vi "BeamGage Callback with notification.vi"(4 "User Parameter":T1, 6 "Control Ref":refnum<k24>, 7 "Event Common Data":T2) -> ()   [LabVIEW 2011]
doc: "A .net callback VI that queries BeamGage for Divergence measurements. Divergence results are loaded into a notifier queue than can be read by an upper level VI as new results become available."
uses:
  C:/Program Files/Spiricon/BeamGage Professional/Spiricon.BeamGage.Automation.Interfaces.dll
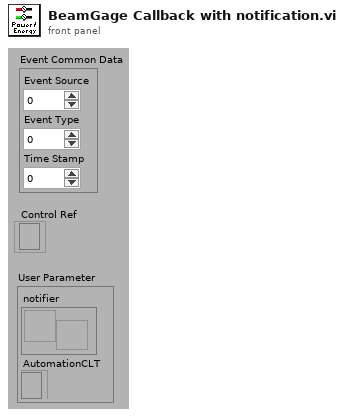
[diagram p1: front panel]
types:
  T1 = cluster{"notifier":refnum<notifier>, "AutomationCLT":refnum<k24>}
  T2 = cluster{"Event Source":i32, "Event Type":u32, "Time Stamp":u32}
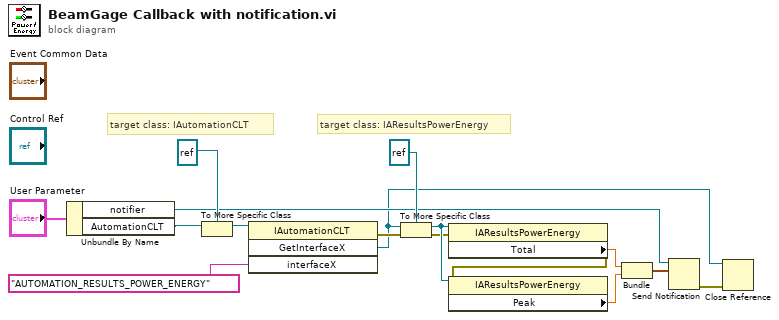
[diagram p0: block diagram]
diagram:
  # "target class: IAResultsPowerEnergy"
  # "target class: IAutomationCLT"
  n1 = Unbundle By Name("User Parameter") -> ("notifier"=w3:refnum<notifier>, "AutomationCLT"=w9:refnum<k24>)
  n2 = To More Specific Class(target class=refnum<k24> refnum, reference=w9) -> (specific class reference=w8:refnum<k24>)  [unwired: 1 in, 1 out]
  n3 = invoke class="IAutomationCLT" method="GetInterfaceX"(reference=w8, "interfaceX"="AUTOMATION_RESULTS_POWER_ENERGY") -> (error out=w11:errorcluster, "GetInterfaceX"=w1:refnum<k24>)  [unwired: 2 in, 2 out]
  n4 = To More Specific Class(target class=refnum<k24> refnum, reference=w1, error in=w11) -> (specific class reference=w15:refnum<k24>, error out=w13:errorcluster)
  n5 = property class="IAResultsPowerEnergy"(reference=w15, error in=w13) -> (error out=w14:errorcluster, "Total"=w6:dbl)  [unwired: 1 out]
  n6 = property class="IAResultsPowerEnergy"(reference=w15, error in=w14) -> ("Peak"=w5:dbl)  [unwired: 2 out]
  n7 = Bundle("Total"=w6, "Peak"=w5) -> (w4:cluster{"Total":dbl, "Peak":dbl})  [unwired: 1 in]
  n8 = Send Notification(notification=w4, notifier=w3) -> (error out=w2:errorcluster)  [unwired: 1 in, 1 out]
  n9 = Close Reference(reference=w1, error in (no error)=w2) -> ()  [unwired: 1 out]
